vi "Test_Target Refresh.vi"() -> ()   [LabVIEW 2019]
uses:
  Build/Project.Dependencies Finder.lvlibp
panel:
  out "Success? Array":bool[](array[boolean])
  out "All Success?":bool
  out "Error Out":errorcluster
  in  "Error In":errorcluster
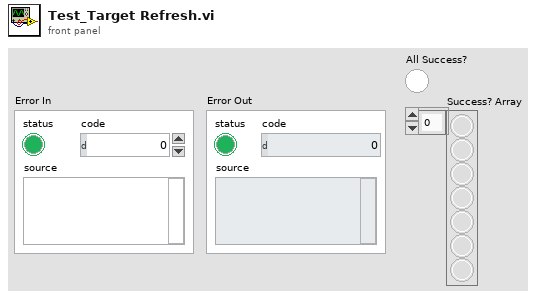
[diagram p1: front panel]
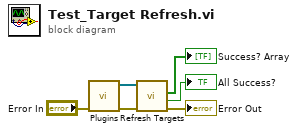
[diagram p0: block diagram]
diagram:
  n1 = call "Plugins.vi"() -> ("Array"=w5:refnum<class "Dependency Source.lvclass">[])  [unwired: 11 in]
  n2 = call "Refresh Targets.vi"("Error In"="Error In", "Dependency Source Plugins"=w5) -> ("Error Out"=→"Error Out":errorcluster, "All Success?"=→"All Success?":bool, "Success? Array"=→"Success? Array":bool[])  [unwired: 7 in]
